vi "FunctDataMgr.Reference Controls.vi"(5 "UUTProps":refnum<vi>, 6 "Vars":refnum<vi>, 7 "SWItems":refnum<vi>, 8 "error in (no error)":errorcluster, 10 "Ctrls.MeasData":refnum<vi>, 11 "FunctDataMgr in":refnum<class "FunctDataMgr.lvclass">) -> (0 "error out":errorcluster, 3 "FunctDataMgr":refnum<class "FunctDataMgr.lvclass">)   [LabVIEW 2018, in "FunctDataMgr.lvclass"]
uses:
  FunctDataMgr.lvclass
  FunctDataMgr.lvclass/FunctDataMgr.ctl
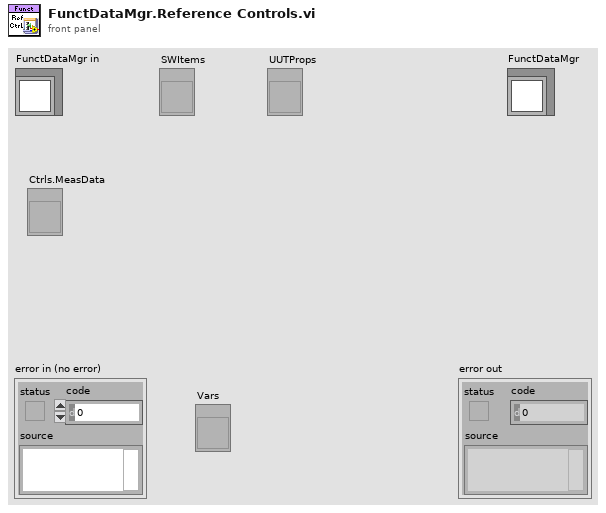
[diagram p1: front panel]
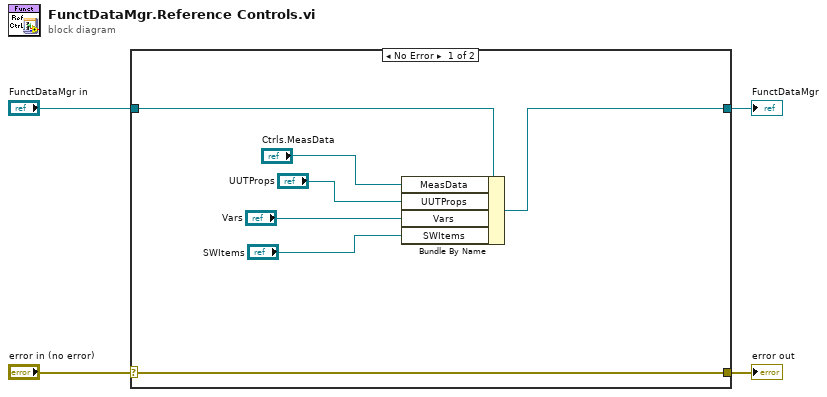
[diagram p0: block diagram]
diagram:
  n1 = case shown="No Error" "error in (no error)" {
    selector: "error in (no error)" -> [w11 w13]
    tunnel: [w11 w13] -> w3
    tunnel: [w9 w12] -> w1
    tunnel: "FunctDataMgr in" -> [w10 w12]
    frame No Error {
      n2 = Bundle By Name(cluster=w10, "MeasData"="Ctrls.MeasData", "UUTProps"="UUTProps", "Vars"="Vars", "SWItems"="SWItems") -> (w9:refnum<class "FunctDataMgr.lvclass">)
    }
    frame Error {
    }
  }
  "error out" <- w3
  "FunctDataMgr" <- w1
